vi "GT Get Gear Ratio.vi"(0 "cardNum":i16, 1 "pMasterSlope":i32, 5 "profile":i16, 7 "pMasterEven":i32, 9 "pSlaveEven":i32, 11 "error in (no error)":errorcluster caption="错误输入（无错误）") -> (3 "pMasterSlope out":i32, 4 "function return":i16, 8 "pMasterEven out":i32, 10 "pSlaveEven out":i32, 15 "error out":errorcluster caption="错误输出")   [LabVIEW 2020, in "gts.lvlib"]
doc: "GT_API GT_GetGearRatio(short cardNum,short profile,long *pMasterEven,long *pSlaveEven,long *pMasterSlope=NULL);"
uses:
  gts.lvlib
  dll/32bit/multi_card/gts.dll
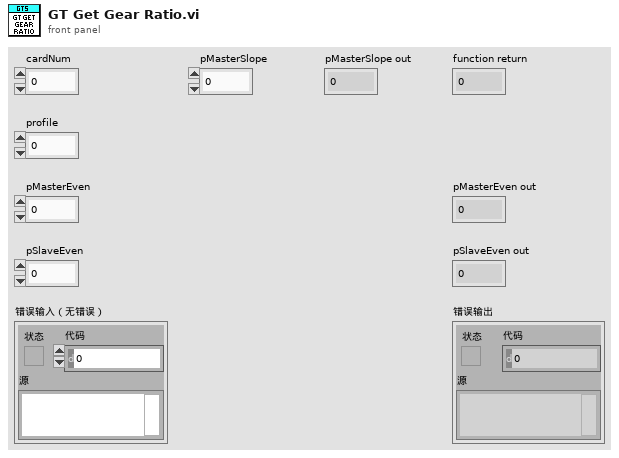
[diagram p1: front panel]
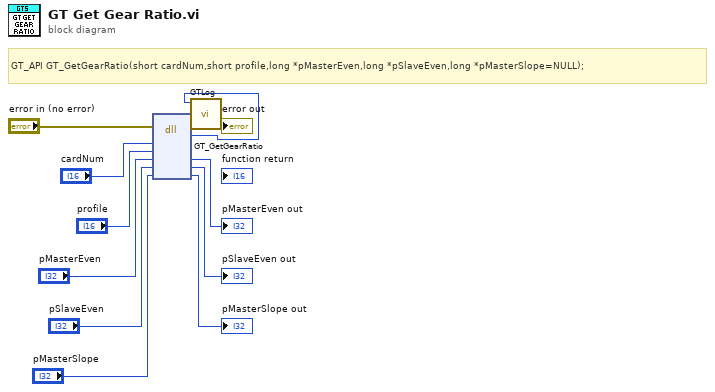
[diagram p0: block diagram]
diagram:
  # "GT_API GT_GetGearRatio(short cardNum,short profile,long *pMasterEven,long *pSlaveEven,long *pMasterSlope=NULL);"
  n1 = dll-call lib="C:/1228/dll/32bit/multi_card/gts.dll" fn="GT_GetGearRatio"(error in="error in (no error)", "cardNum"="cardNum", "profile"="profile", "pMasterEven"="pMasterEven", "pSlaveEven"="pSlaveEven", "pMasterSlope"="pMasterSlope") -> (error out=w3:errorcluster, w1:i16, "pMasterEven"=→"pMasterEven out":i32, "pSlaveEven"=→"pSlaveEven out":i32, "pMasterSlope"=→"pMasterSlope out":i32)  [unwired: 4 in, 1 out]
  n2 = call "GTLog.vi"("error in (no error)"=w3, "Numeric"=w1) -> ("error out"=→"error out":errorcluster)  [unwired: 9 in]
